vi "ManagerTcpSample.vi"() -> ()   [LabVIEW 2021]
doc: "マネージャーPC用TCP通信サンプル"
uses:
  SubVI/TcpCommunicationServerData.ctl
  SubVI/HallMeasurementStatus.ctl
  SubVI/TcpCommunicationServerCMD.ctl
panel:
  in  "Tab Control":enum32{"Test"}(tab)
  in  "H_Status":bool
  in  "Sample Name":string="Sample"
  in  "H_Placed":bool
  in  "Setting File Path":path=path "Setting"
  in  "H_Setting":bool
  in  "H_Start":bool
  in  "H_Data":bool
  in  "H_Collected":bool
  in  "TestPCアドレス":string="192.168.1.114" caption="Address"
  out "TestData":T2
  out "Read Log":T3(array[cluster])
  out "接続数":i32
  out "Send List":cluster{"Address":string, "Data":string}[](array[cluster])
  out "Data":T4
  in  "ポート":u16=8501
  in  "停止":bool
  # "マネージャーPC用TCP通信サンプル"
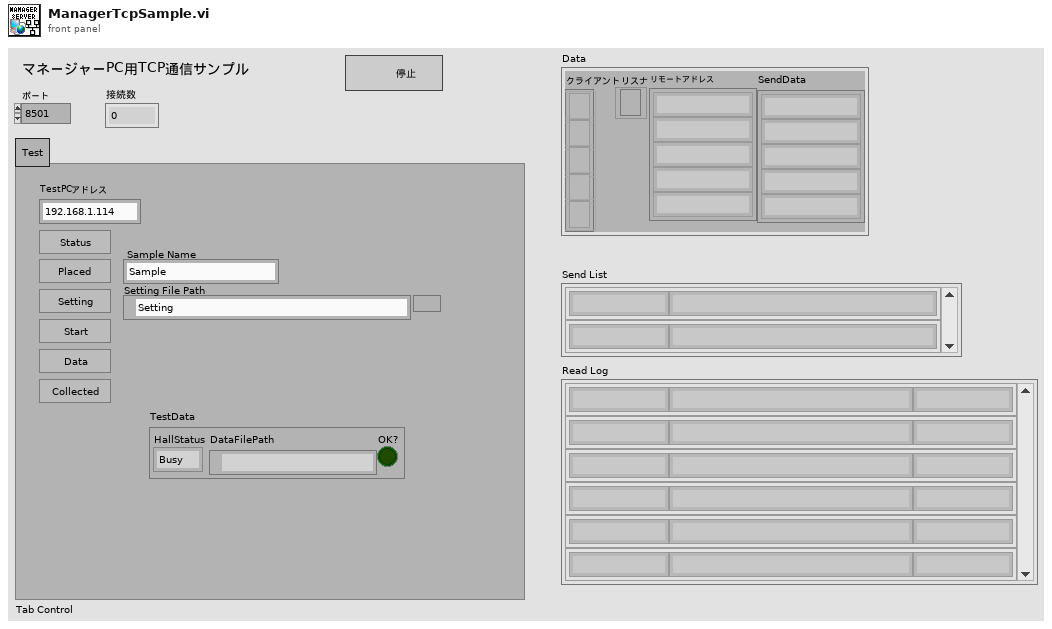
[diagram p1: front panel]
types:
  T1 = typedef "HallMeasurementStatus.ctl" = enum16{"Busy", "Ready", "Done", "Error"}
  T2 = cluster{"HallStatus":T1, "DataFilePath":path, "OK?":bool}
  T3 = cluster{"Address":string, "Data":string, "SendData":string}[]
  T4 = typedef "TcpCommunicationServerData.ctl" = cluster{"クライアント":refnum<k5>[], "リスナ":refnum<k5>, "リモートアドレス":string[], "SendData":string[]}
  T5 = typedef "TcpCommunicationServerCMD.ctl" = enum16{"Initialize", "Status Check", "Send Data", "Read Data", "Stop", "GetData"}
  T6 = typedef "TestMeasurementStatus.ctl" = enum16{"Busy", "Ready", "Done", "Error"}
  T7 = cluster{"Status":T6, "DataFilePath":path, "OK?":bool}
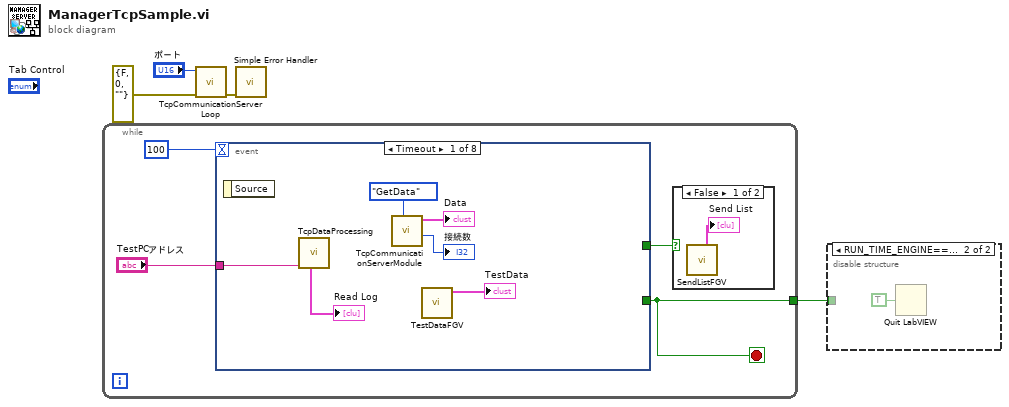
[diagram p0: block diagram]
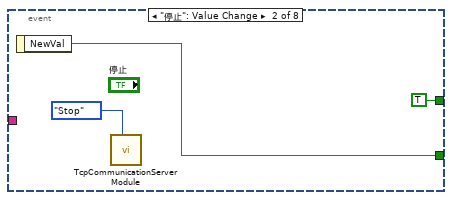
[diagram p4: hidden frame]
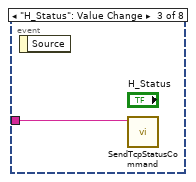
[diagram p5: hidden frame]
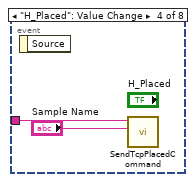
[diagram p6: hidden frame]
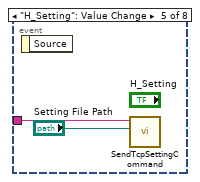
[diagram p7: hidden frame]
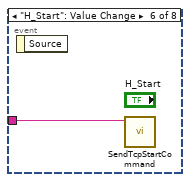
[diagram p8: hidden frame]
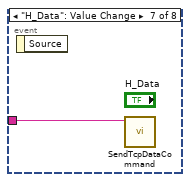
[diagram p9: hidden frame]
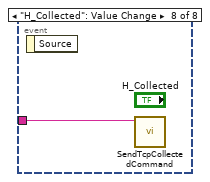
[diagram p10: hidden frame]
diagram:
  n1 = while {
    tunnel: [w5] -> w1
    stop <- w5 stop-if-true
    n2 = event shown="[0] Timeout" {
      selector: _ -> [_ _ _ _ _ _ _ _]
      dyn-events: _ -> [_ _ _ _ _ _ _ _]
      timeout: 100 -> [_ _ _ _ _ _ _ _]
      tunnel: [_ w18 _ _ _ _ _ _] -> w5
      tunnel: "TestPCアドレス" -> [w11 _ w19 w20 w22 w24 w25 w26]
      tunnel: [_ TRUE ("H_Setting") _ _ _ _ _ _] -> w6
      event Timeout {
        n3 = event-data() -> ()  [unwired: 1 in, 1 out]
        n4 = call "TcpDataProcessing.vi"("TestPCアドレス"=w11) -> ("Read Log"=→"Read Log":T3)  [unwired: 9 in, 1 out]
        n5 = call "TcpCommunicationServerModule.vi"("States"=TcpCommunicationServerCMD."GetData") -> ("接続数"=→"接続数":i32, "Data出力"=→"Data":T4)  [unwired: 7 in, 2 out]
        n6 = call "TestDataFGV.vi"() -> ("TestData Out"=→"TestData":T7)  [unwired: 11 in]
      }
      event "停止": Value Change {
        n7 = event-data() -> ("NewVal"=w18:bool)  [unwired: 1 in]
        n8 = call "TcpCommunicationServerModule.vi"("States"=TcpCommunicationServerCMD."Stop") -> ()  [unwired: 7 in, 4 out]
      }
      event "H_Status": Value Change {
        n9 = event-data() -> ()  [unwired: 1 in, 1 out]
        n10 = call "SendTcpStatusCommand.vi"("アドレス"=w19) -> ()  [unwired: 8 in, 3 out]
      }
      event "H_Placed": Value Change {
        n11 = event-data() -> ()  [unwired: 1 in, 1 out]
        n12 = call "SendTcpPlacedCommand.vi"("Sample Name"="Sample Name", "アドレス"=w20) -> ()  [unwired: 7 in, 3 out]
      }
      event "H_Setting": Value Change {
        n13 = event-data() -> ()  [unwired: 1 in, 1 out]
        n14 = call "SendTcpSettingCommand.vi"("Setting File Path"="Setting File Path", "アドレス"=w22) -> ()  [unwired: 7 in, 3 out]
      }
      event "H_Start": Value Change {
        n15 = event-data() -> ()  [unwired: 1 in, 1 out]
        n16 = call "SendTcpStartCommand.vi"("アドレス"=w24) -> ()  [unwired: 8 in, 3 out]
      }
      event "H_Data": Value Change {
        n17 = event-data() -> ()  [unwired: 1 in, 1 out]
        n18 = call "SendTcpDataCommand.vi"("アドレス"=w25) -> ()  [unwired: 8 in, 3 out]
      }
      event "H_Collected": Value Change {
        n19 = event-data() -> ()  [unwired: 1 in, 1 out]
        n20 = call "SendTcpCollectedCommand.vi"("アドレス"=w26) -> ()  [unwired: 8 in, 3 out]
      }
    }
    n21 = case shown="False" w6 {
      frame False {
        n22 = call "SendListFGV.vi"() -> ("Send List Out"=→"Send List":cluster{"Address":string, "Data":string}[])  [unwired: 9 in, 2 out]
      }
      frame True {
      }
    }
  }
  n23 = call "TcpCommunicationServerLoop.vi"("エラー入力（エラーなし）"=errorcluster {"status"=FALSE, "code"=0, "source"=""} ("error constant"), "ポート"="ポート") -> ("エラー出力"=w3:errorcluster)  [unwired: 9 in]
  n24 = call <vilib>:"Simple Error Handler.vi"("error in (no error)"=w3) -> ()  [unwired: 4 in, 5 out]
  n25 = disable-structure shown="RUN_TIME_ENGINE==True" {
    disable-tunnel: w1 -> [_ _]
    frame condition #0 (active) {
    }
    frame condition #1 {
      n26 = Quit LabVIEW(quit? (T)=TRUE) -> ()
    }
  }
